vi "GreeterService SayHello.vi"(3 "error in (no error)":errorcluster, 4 "gRPCid in":T1, 5 "DNL_LabVIEW Object in":refnum<class "GreeterServiceImpl.lvclass">) -> (0 "error out":errorcluster, 1 "gRPCid out":T1, 2 "DNL_LabVIEW Object out":refnum<class "GreeterServiceImpl.lvclass">)   [LabVIEW 2019, in "UserCode_server.lvlib" / "GreeterServiceImpl.lvclass"]
uses:
  GreeterServiceImpl.lvclass
  <vilib>/gRPC/LabVIEW gRPC Library/Shared/grpcId.ctl
  Generated_server/RPC Service/GreeterService/GreeterService.lvclass
  <vilib>/gRPC/LabVIEW gRPC Library/grpc-lvsupport-release.lvlib
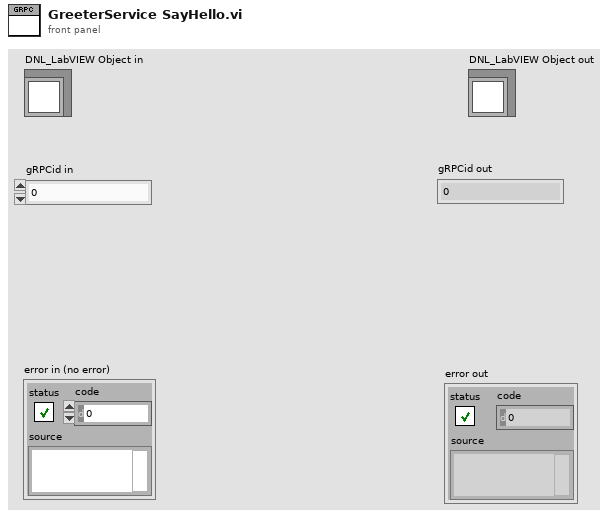
[diagram p1: front panel]
types:
  T1 = typedef "grpc-lvsupport-release.lvlib/grpcId.ctl" = u64
  T2 = typedef "Generated_server.lvlib/helloworld_HelloRequest.ctl" = cluster{"name":string}
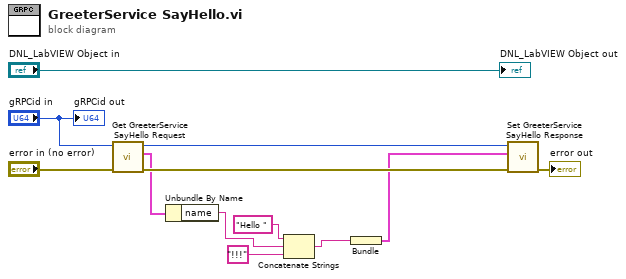
[diagram p0: block diagram]
diagram:
  n1 = call "Get GreeterService SayHello Request.vi"("error in (no error)"="error in (no error)", "gRPCid"="gRPCid in") -> ("error out"=w10:errorcluster, "Message Data"=w5:T2, "gRPCid out"=w7:T1)  [unwired: 7 in]
  n2 = Unbundle By Name(w5) -> ("name"=w4:string)
  n3 = Concatenate Strings("Hello ", w4, "!!!") -> (w2:string)
  n4 = Bundle(w2) -> (w1:cluster{string})  [unwired: 1 in]
  n5 = call "Set GreeterService SayHello Response.vi"("error in (no error)"=w10, "Message Data"=w1, "gRPCid in"=w7) -> ("error out"=→"error out":errorcluster)  [unwired: 8 in]
  "DNL_LabVIEW Object out" <- "DNL_LabVIEW Object in"
  "gRPCid out" <- "gRPCid in"
